vi "Actor Core.vi"(8 "error in":errorcluster, 11 "Member_Actor in":refnum<class "Member_Actor.lvclass">) -> (0 "error out":errorcluster, 3 "Actor out":refnum<class "Actor.lvclass">)   [LabVIEW 2015, in "Member_Actor.lvlib" / "Member_Actor.lvclass"]
doc: "(<B>Filename</B>: Actor Framework.lvlib:Actor.lvclass:Actor Core.vi)\n\nReceives messages to the actor, reacts to them, and initiates any error handling that may shut the actor down.\n\nDescendant classes may override this VI to append parallel tasks for the actor to complete while it handles messages. Overrides use the Call Parent Method node."
uses:
  Member_Actor.lvclass
  <vilib>/ActorFramework/Actor/Actor.lvclass
  <vilib>/ActorFramework/Actor/Actor.lvclass/Actor.ctl
  <vilib>/ActorFramework/Message Enqueuer/Message Enqueuer.lvclass/Message Enqueuer.ctl
  <vilib>/ActorFramework/Message Enqueuer/Init from Existing Queue.vi
  User_Actor/User_Actor/User_Actor.lvclass
  <vilib>/ActorFramework/Message Enqueuer/Message Enqueuer.lvclass
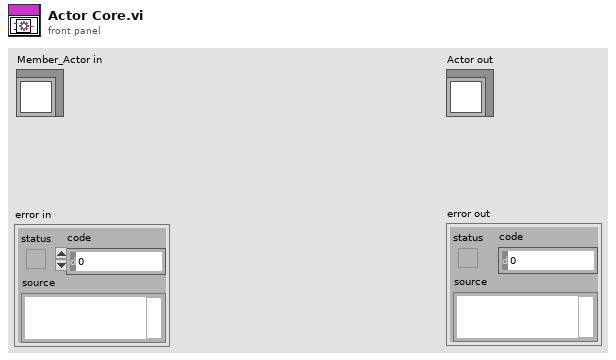
[diagram p1: front panel]
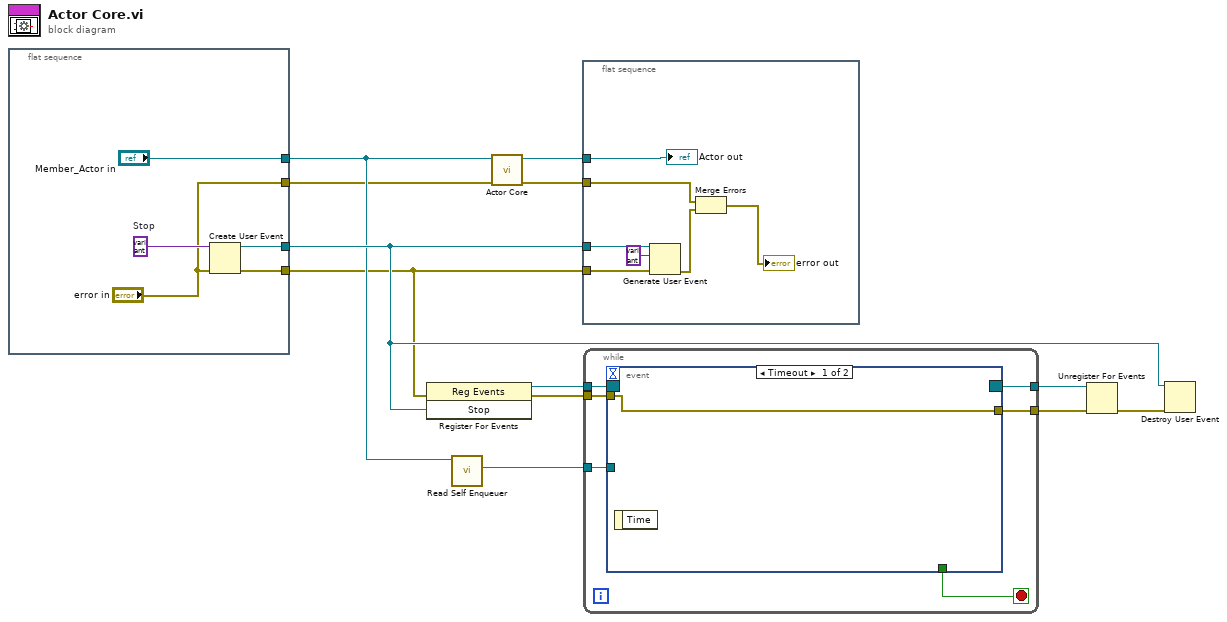
[diagram p0: block diagram]
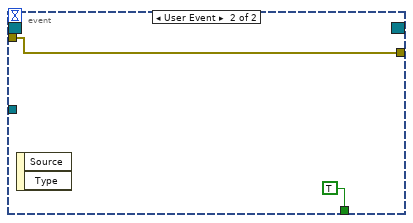
[diagram p2: hidden frame]
diagram:
  n1 = flat-sequence {
    tunnel: ["error in"] -> w3
    tunnel: ["Member_Actor in"] -> w7
    tunnel: [w16] -> w11
    tunnel: [w15] -> w5
    frame #0 {
      w17 = variant  # Stop
      n2 = Create User Event(user event datatype=w17, error in="error in") -> (user event=w16:refnum<user-event>, error out=w15:errorcluster)
    }
  }
  n3 = register-events(error in=w5, w11) -> (reference out=w4:refnum<event-registration>, error out=w6:errorcluster)  [unwired: 1 in]
  n4 = call <vilib>:"Read Self Enqueuer.vi"("Actor"=w7) -> ("Self Enqueuer"=w8:refnum<class "Message Enqueuer.lvclass">)  [unwired: 10 in]
  n5 = call-parent "Actor Core.vi"("error in"=w3, "Actor in"=w7) -> ("error out"=w1:errorcluster, "Actor out"=w2:refnum<class "Actor.lvclass">)  [unwired: 8 in]
  n6 = flat-sequence {
    tunnel: w1 -> [w20]
    tunnel: w2 -> [w21]
    tunnel: w11 -> [w24]
    tunnel: w5 -> [w23]
    frame #0 {
      n7 = Generate User Event(user event=w24, event data cluster=variant ("event data"), error in=w23) -> (error out=w19:errorcluster)  [unwired: 1 in, 1 out]
      n8 = Merge Errors(w20, w19) -> (→"error out":errorcluster)
      "Actor out" <- w21
    }
  }
  n9 = while {
    tunnel: w4 -> [w30]
    tunnel: w6 -> [w29]
    tunnel: w8 -> [w28]
    tunnel: [w26] -> w9
    tunnel: [w25] -> w10
    stop <- w27 stop-if-true
    n10 = event shown="[0] Timeout" {
      selector: w30 -> [_ _]
      dyn-events: [_ _] -> w26
      timeout: _ -> [_ _]
      tunnel: w29 -> [w31 w32]
      tunnel: w28 -> [_ _]
      tunnel: [_ TRUE] -> w27
      tunnel: [w31 w32] -> w25
      event Timeout {
        n11 = event-data() -> ()  [unwired: 1 in, 1 out]
      }
      event User Event {
        n12 = event-data() -> ()  [unwired: 1 in, 2 out]
      }
    }
  }
  n13 = Unregister For Events(event registration refnum=w9, error in=w10) -> (error out=w12:errorcluster)
  n14 = Destroy User Event(user event=w11, error in=w12) -> ()  [unwired: 1 out]
